vi "Reset.vi"(8 "error in":errorcluster, 11 "4124 in":refnum<class "4124.lvclass">) -> (0 "error out":errorcluster, 3 "4124 out":refnum<class "4124.lvclass">)   [LabVIEW 2018, in "4124.lvlib" / "4124.lvclass"]
uses:
  4124.lvclass
  builds/Power_Supply.lvlibp/Power Supply.lvclass
  <instrlib>/NI RMX-412x Power Supplies/NI RMX-412x Power Supplies.lvlib
  C:/Users/Ron.Dexter.LUMINARTECH/Desktop/builds/Power_Supply.lvlibp/Power Supply.lvclass
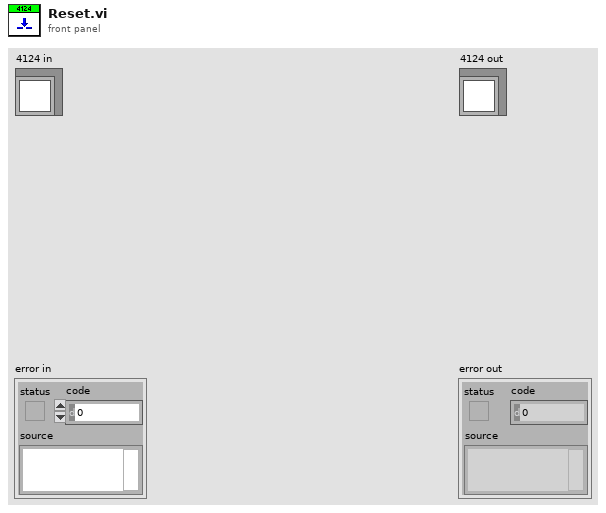
[diagram p1: front panel]
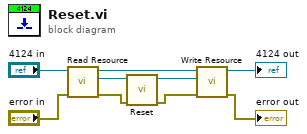
[diagram p0: block diagram]
diagram:
  n1 = call "Read Resource.vi"("error in"="error in", "Power Supply in"="4124 in") -> ("error out"=w3:errorcluster, "Resource"=w5:refnum<visa-resource-name>, "Power Supply out"=w7:refnum<class "4124.lvclass">)  [unwired: 7 in]
  n2 = call <instrlib>:"Reset.vi"("error in (no error)"=w3, "VISA resource name"=w5) -> ("error out"=w2:errorcluster, "VISA resource name out"=w4:refnum<visa-resource-name>)  [unwired: 8 in]
  n3 = call "Write Resource.vi"("error in"=w2, "Resource"=w4, "Power Supply in"=w7) -> ("error out"=→"error out":errorcluster, "Power Supply out"=→"4124 out":refnum<class "4124.lvclass">)  [unwired: 7 in]
